vi "Compute Linear Coefficients.vi"(8 "Error In":errorcluster, 9 "Point 2":cluster{"X":dbl, "Y":dbl}, 11 "Point 1":cluster{"X":dbl, "Y":dbl}) -> (0 "Error Out":errorcluster, 3 "Linear Coefficients":cluster{"u":dbl, "v":dbl})   [LabVIEW 2019]
uses:
  <vilib>/Utility/error.llb/Error Cluster From Error Code.vi
  <vilib>/ErrorRing/Error Ring.xnode
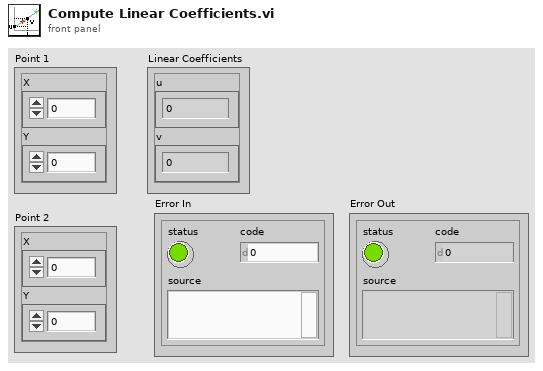
[diagram p1: front panel]
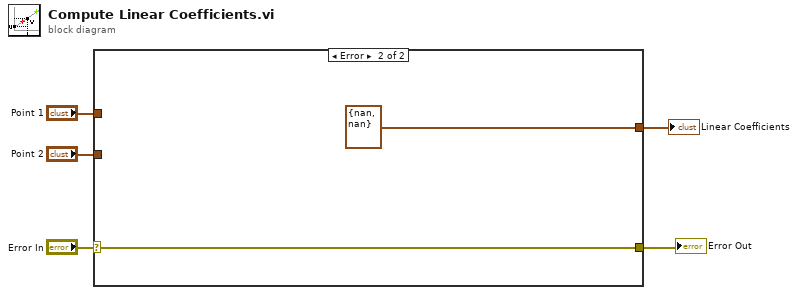
[diagram p0: block diagram]
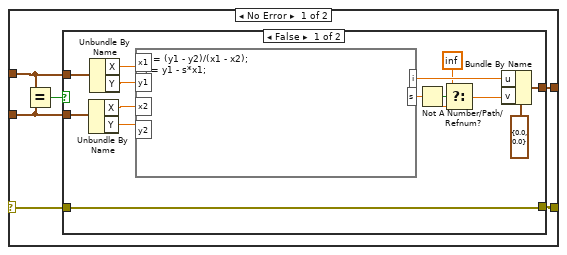
[diagram p2: hidden frame]
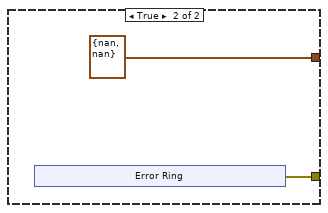
[diagram p3: hidden frame]
diagram:
  n1 = case shown="Error" "Error In" {
    selector: "Error In" -> [w6 w33]
    tunnel: "Point 1" -> [w9 _]
    tunnel: "Point 2" -> [w8 _]
    tunnel: [w10 w33] -> w2
    tunnel: [w7 cluster{"u":dbl, "v":dbl} {"u"=nan, "v"=nan} ("Linear Coefficients")] -> w1
    frame No Error {
      n2 = Equal?(x=w9, y=w8) -> (x = y?=w11:bool)
      n3 = case shown="False" w11 {
        tunnel: [w14 w27] -> w10
        tunnel: w9 -> [w25 _]
        tunnel: w8 -> [w24 _]
        tunnel: [w12 cluster{"u":dbl, "v":dbl} {"u"=nan, "v"=nan} ("Linear Coefficients")] -> w7
        tunnel: w6 -> [w14 _]
        frame False {
          n4 = Unbundle By Name(w24) -> ("X"=w20:dbl, "Y"=w19:dbl)
          n5 = Unbundle By Name(w25) -> ("X"=w22:dbl, "Y"=w21:dbl)
          n6 = formula code="s = (y1 - y2)/(x1 - x2);\ni = y1 - s*x1;"("x1"=w22, "y1"=w21, "x2"=w20, "y2"=w19) -> ("i"=w23:dbl, "s"=w15:dbl)
          n7 = Not A Number/Path/Refnum?(number/path/refnum=w15) -> (NaN/Path/Refnum?=w18:bool)
          n8 = Select(t=inf, s=w18, f=w15) -> (s? t:f=w17:dbl)
          n9 = Bundle By Name(cluster=cluster{"u":dbl, "v":dbl} {"u"=0.0, "v"=0.0} ("Linear Coefficients"), "u"=w23, "v"=w17) -> (w12:cluster{"u":dbl, "v":dbl})
        }
        frame True {
          n10 = xnode "Error Ring"() -> ("error out"=w27:errorcluster)
        }
      }
    }
    frame Error {
    }
  }
  "Linear Coefficients" <- w1
  "Error Out" <- w2
